vi "PoseAndTargeting.vi"() -> ()   [LabVIEW 2019]
doc: "This VI manages the robot's pose (position, heading, and velocity) and targeting information. Data from the IMU, swerve drive encoders, swerve azimuth encoders, LimeLight, and LIDAR are fused together to estimate these values. Supports pose resets on boot, from the Autonomous Sequencer, and on command from the FRC 4265 Dashboard."
uses:
  dsinstructions.vi
  sensors.vi
  dsdata.vi
  outputs.vi
  constants.vi
  autoninfo.vi
panel:
  out "Y Position (in)":dbl
  out "X Position (in)":dbl
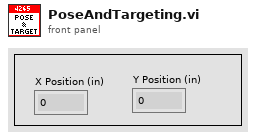
[diagram p1: front panel]
types:
  T1 = enum16{"Center", "North", "NorthWest", "West", "SouthWest", "South", "SouthEast", "East", "NorthEast"}
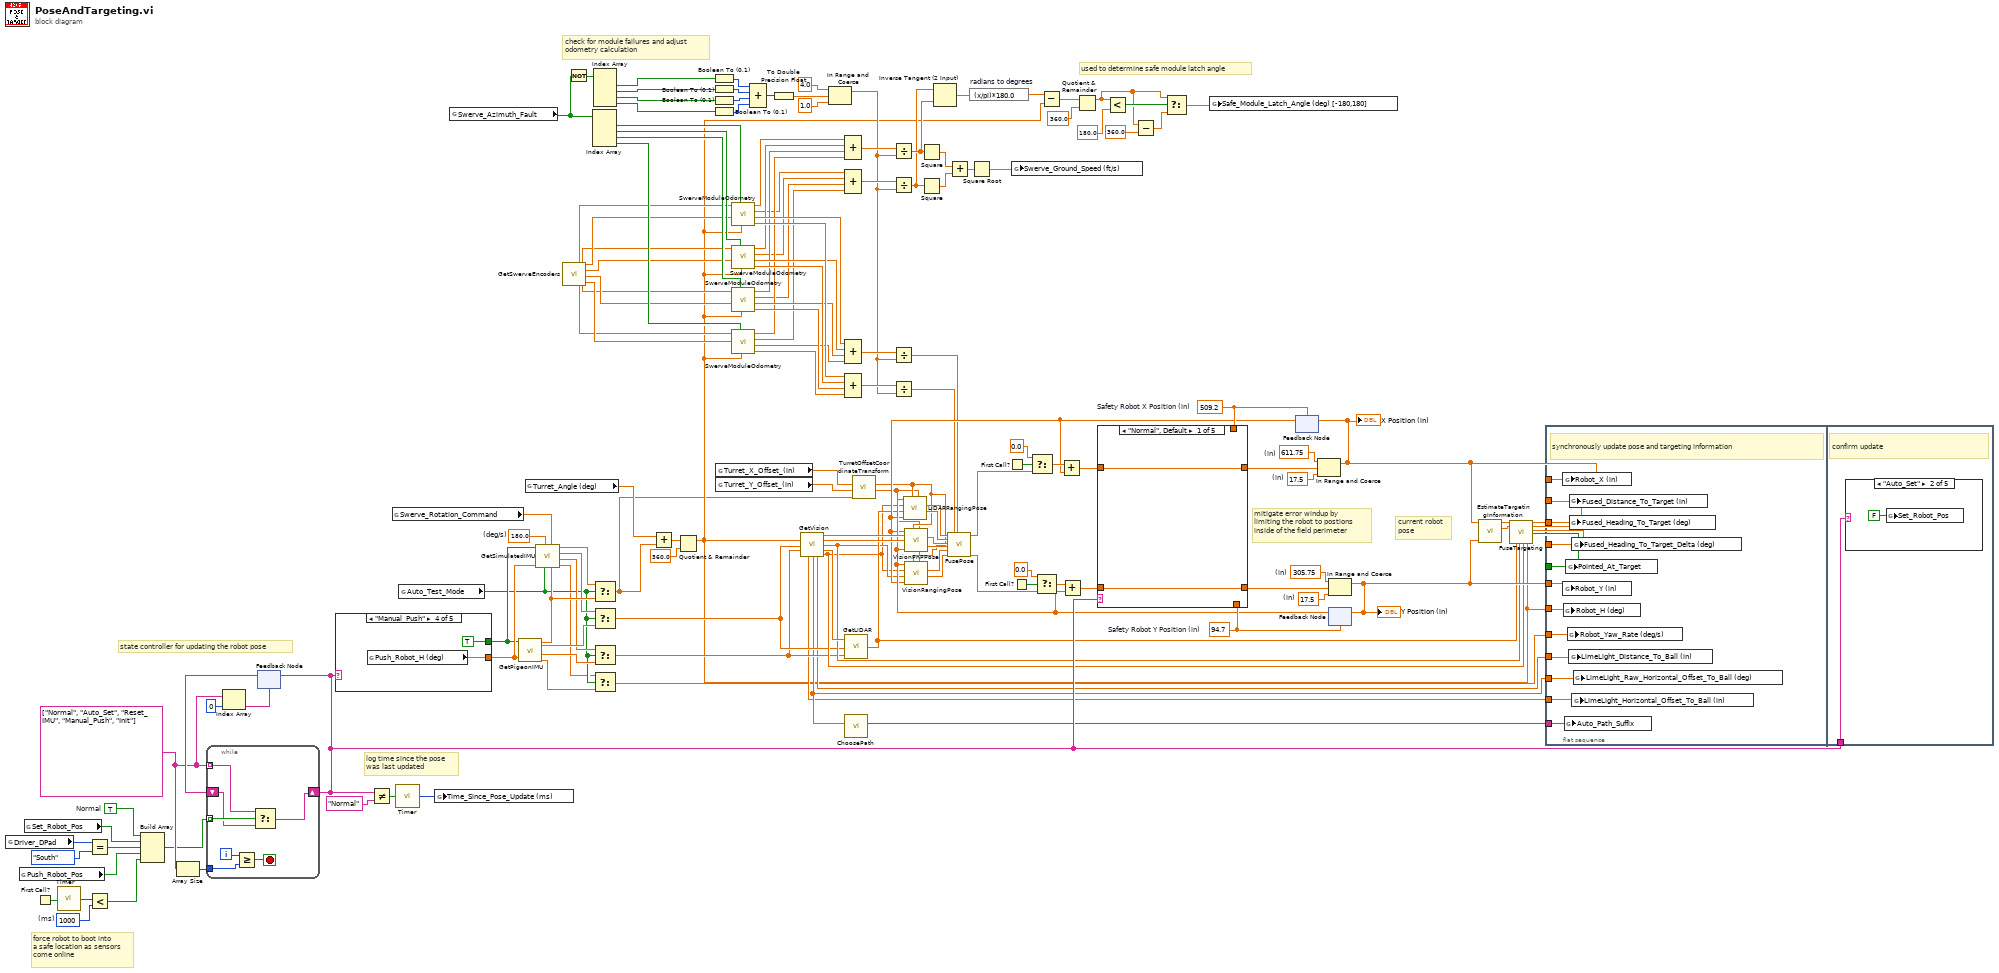
[diagram p0: block diagram]
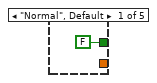
[diagram p6: hidden frame]
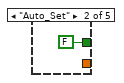
[diagram p7: hidden frame]
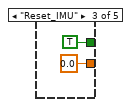
[diagram p8: hidden frame]
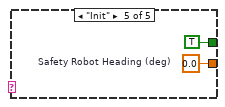
[diagram p9: hidden frame]
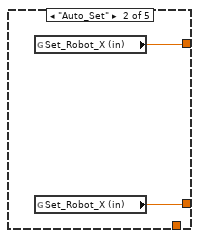
[diagram p10: hidden frame]
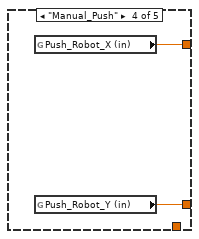
[diagram p12: hidden frame]
diagram:
  w94 = 180.0  # (deg/s)
  w98 = u32 1000  # (ms)
  w116 = string[] ["Normal", "Auto_Set", "Reset_IMU", "Manual_Push", "Init"] ("State Names")
  w115 = TRUE  # Normal
  w125 = 305.75  # (in)
  w126 = 17.5  # (in)
  w130 = 611.75  # (in)
  w131 = 17.5  # (in)
  w103 = 509.2  # Safety Robot X Position (in)
  w102 = 94.7  # Safety Robot Y Position (in)
  # "used to determine safe module latch angle"
  # "force robot to boot into\na safe location as sensors\ncome online"
  # "log time since the pose\nwas last updated"
  # "state controller for updating the robot pose"
  # "current robot\npose"
  # "mitigate error windup by\nlimiting the robot to postions\ninside of the field perimeter"
  # "check for module failures and adjust\nodometry calculation"
  n1 = global read "dsinstructions.vi" "Driver_DPad"() -> (w133:T1)
  n2 = global read "sensors.vi" "Push_Robot_Pos"() -> (w117:bool)
  n3 = global read "sensors.vi" "Set_Robot_Pos"() -> (w93:bool)
  n4 = First Call?() -> (First Call?: T/F=w101:bool)
  n5 = call "Timer.vi"("Reset Timer"=w101) -> ("Time (ms)"=w100:u32)
  n6 = Equal?(x=w133, y=T1."South") -> (x = y?=w92:bool)
  n7 = Less?(x=w100, y=w98) -> (x < y?=w99:bool)
  n8 = Build Array(w115, w93, w92, w117, w99) -> (w114:bool[])
  n9 = Array Size(array=w116) -> (size(s)=w118:i32)
  n10 = Index Array(array=w116, index=0) -> (element=w120:string)
  n11 = feedback #1(w120) -> (w119:string)
  n12 = while {
    tunnel: w114 -> [w161] mode=indexing
    tunnel: w116 -> [w159] mode=indexing
    shift-right: [w158] -> w107
    shift-left: w119 -> [w160]
    tunnel: w118 -> [w156]
    i -> [w157]
    stop <- w155 stop-if-true
    n13 = Greater Or Equal?(x=w157, y=w156) -> (x >= y?=w155:bool)
    n14 = Select(t=w159, s=w161, f=w160) -> (s? t:f=w158:string)
  }
  n15 = feedback-in #1(w107) -> ()
  n16 = case shown="\"Manual_Push\"" w107 {
    tunnel: [_ _ 0.0 ("Push_Robot_H (deg)") w167 w168] -> w97
    tunnel: [FALSE FALSE TRUE TRUE TRUE] -> w96
    frame "Normal", Default {
    }
    frame "Auto_Set" {
    }
    frame "Reset_IMU" {
    }
    frame "Manual_Push" {
      n17 = global read "sensors.vi" "Push_Robot_H (deg)"() -> (w167:dbl)
    }
    frame "Init" {
      w168 = 0.0  # Safety Robot Heading (deg)
    }
  }
  n18 = Not Equal?(x=w107, y="Normal") -> (x != y?=w106:bool)
  n19 = global read "outputs.vi" "Swerve_Rotation_Command"() -> (w95:dbl)
  n20 = call "Timer.vi"("Reset Timer"=w106) -> ("Time (ms)"=w104:u32)
  n21 = global read "dsdata.vi" "Auto_Test_Mode"() -> (w25:bool)
  n22 = global write "sensors.vi" "Time_Since_Pose_Update (ms)"(w104) -> ()
  n23 = global read "sensors.vi" "Swerve_Azimuth_Fault"() -> (w148:bool[])
  n24 = call "GetPigeonIMU.vi"("Reset Yaw (deg)"=w97, "Reset Yaw"=w96) -> ("Yaw Rate (deg/s)"=w24:dbl, "Roll (deg)"=w55:dbl, "Pitch (deg)"=w57:dbl, "Yaw (deg)"=w59:dbl)  [unwired: 6 in]
  n25 = global read "sensors.vi" "Turret_Angle (deg)"() -> (w9:dbl)
  n26 = call "GetSimulatedIMU.vi"("Real IMU Yaw (deg)"=w59, "Rotation Command"=w95, "Auto Test Mode"=w25, "Max Simulated Rotation Speed (deg/s)"=w94, "Reset Yaw (deg)"=w97, "Reset Yaw"=w96) -> ("Simulated Yaw Rate (deg/s)"=w23:dbl, "Simulated Roll (deg)"=w56:dbl, "Simulated Pitch (deg)"=w58:dbl, "Simulated Yaw (deg)"=w60:dbl)  [unwired: 2 in]
  n27 = call "GetSwerveEncoders.vi"() -> ("Swerve 0 Velocity (ft/s)"=w33:dbl, "Swerve 3 Velocity (ft/s)"=w30:dbl, "Swerve 1 Velocity (ft/s)"=w32:dbl, "Swerve 2 Velocity (ft/s)"=w31:dbl, "Swerve 0 Azimuth Position (deg)"=w91:dbl, "Swerve 1 Azimuth Position (deg)"=w90:dbl, "Swerve 2 Azimuth Position (deg)"=w89:dbl, "Swerve 3 Azimuth Position (deg)"=w88:dbl)  [unwired: 20 in]
  n28 = Not(x=w148) -> (.not. x?=w147:bool[])
  n29 = Index Array(array=w148) -> (element #1=w137:bool, element #2=w136:bool, element #3=w135:bool, element #4=w134:bool)  [unwired: 4 in]
  n30 = Index Array(array=w147) -> (element #1=w146:bool, element #2=w145:bool, element #3=w144:bool, element #4=w143:bool)  [unwired: 4 in]
  n31 = Select(t=w60, s=w25, f=w59) -> (s? t:f=w3:dbl)
  n32 = Select(t=w58, s=w25, f=w57) -> (s? t:f=w54:dbl)
  n33 = Select(t=w56, s=w25, f=w55) -> (s? t:f=w53:dbl)
  n34 = Select(t=w23, s=w25, f=w24) -> (s? t:f=w22:dbl)
  n35 = Add(x=w9, y=w3) -> (x+y=w8:dbl)
  n36 = Quotient & Remainder(x=w8, y=360.0) -> (x-y*floor(x/y)=w6:dbl)  [unwired: 1 out]
  n37 = Boolean To (0,1)(Boolean=w146) -> (0, 1=w142:i16)
  n38 = Boolean To (0,1)(Boolean=w145) -> (0, 1=w141:i16)
  n39 = Boolean To (0,1)(Boolean=w144) -> (0, 1=w140:i16)
  n40 = Boolean To (0,1)(Boolean=w143) -> (0, 1=w139:i16)
  n41 = global read "constants.vi" "Turret_X_Offset_(in)"() -> (w5:dbl)
  n42 = global read "constants.vi" "Turret_Y_Offset_(in)"() -> (w4:dbl)
  n43 = call "SwerveModuleOdometry.vi"("Robot Heading(deg)"=w6, "Module Fault"=w137, "Wheel Azimuth (deg)"=w91, "Velocity (ft/s)"=w33) -> ("Delta Y (in)"=w149:dbl, "Delta X (in)"=w52:dbl, "Velocity Y (ft/s)"=w44:dbl, "Velocity X (ft/s)"=w48:dbl)  [unwired: 2 in]
  n44 = call "SwerveModuleOdometry.vi"("Robot Heading(deg)"=w6, "Module Fault"=w136, "Wheel Azimuth (deg)"=w90, "Velocity (ft/s)"=w32) -> ("Delta Y (in)"=w150:dbl, "Delta X (in)"=w51:dbl, "Velocity Y (ft/s)"=w43:dbl, "Velocity X (ft/s)"=w47:dbl)  [unwired: 2 in]
  n45 = call "SwerveModuleOdometry.vi"("Robot Heading(deg)"=w6, "Module Fault"=w135, "Wheel Azimuth (deg)"=w89, "Velocity (ft/s)"=w31) -> ("Delta Y (in)"=w151:dbl, "Delta X (in)"=w50:dbl, "Velocity Y (ft/s)"=w42:dbl, "Velocity X (ft/s)"=w46:dbl)  [unwired: 2 in]
  n46 = call "SwerveModuleOdometry.vi"("Robot Heading(deg)"=w6, "Module Fault"=w134, "Wheel Azimuth (deg)"=w88, "Velocity (ft/s)"=w30) -> ("Delta Y (in)"=w152:dbl, "Delta X (in)"=w49:dbl, "Velocity Y (ft/s)"=w41:dbl, "Velocity X (ft/s)"=w45:dbl)  [unwired: 2 in]
  n47 = Compound Arithmetic op=ADD(w142, w141, w140, w139) -> (w138:i16)
  n48 = To Double Precision Float(number=w138) -> (double precision float=w83:dbl)
  n49 = call "GetVision.vi"("Turret_H (deg)"=w6, "Pitch (deg)"=w54, "Roll (deg)"=w53) -> ("LimeLight Raw Z Power Port (in)"=w87:dbl, "LimeLight Raw X Power Port (in)"=w86:dbl, "LimeLight Distance to Power Port (in)"=w66:dbl, "LimeLight Raw Horizontal Offset Power Port (deg)"=w68:dbl, "LimeLight Horizontal Offset to Ball (in)"=w26:dbl, "LimeLight Raw Horizontal Offset to Ball (deg)"=w28:dbl, "LimeLight Distance to Ball (in)"=w29:dbl, "LimeLight Heading to Power Port (deg)"=w61:dbl)  [unwired: 5 in]
  n50 = In Range and Coerce(upper limit=4.0, x=w83, lower limit=1.0) -> (coerced(x)=w38:dbl)  [unwired: 1 out]
  n51 = Compound Arithmetic op=ADD(w48, w47, w46, w45) -> (w40:dbl)
  n52 = Compound Arithmetic op=ADD(w44, w43, w42, w41) -> (w39:dbl)
  n53 = Compound Arithmetic op=ADD(w52, w51, w50, w49) -> (w154:dbl)
  n54 = Compound Arithmetic op=ADD(w149, w150, w151, w152) -> (w153:dbl)
  n55 = call "GetLIDAR.vi"("Roll (deg)"=w53, "Pitch (deg)"=w54, "Raw Horizontal Offset (in)"=w68) -> ("LIDAR Distance to Target (in)"=w67:dbl)
  n56 = call "ChoosePath.vi"("Limelight Raw Horizontal Offset to Ball (deg)"=w28) -> ("Auto Path Suffix"=w27:string)  [unwired: 10 in]
  n57 = call "TurretOffsetCoordinateTransform.vi"("Robot_Heading_(deg)"=w3, "Turret_Y_Offset_(in)"=w4, "Turret_X_Offset_(in)"=w5) -> ("Turret_Delta_Y"=w1:dbl, "Turret_Delta_X"=w2:dbl)  [unwired: 7 in]
  n58 = Divide(x=w40, y=w38) -> (x/y=w21:dbl)
  n59 = Divide(x=w39, y=w38) -> (x/y=w20:dbl)
  n60 = Divide(x=w154, y=w38) -> (x/y=w78:dbl)
  n61 = Divide(x=w153, y=w38) -> (x/y=w77:dbl)
  n62 = Square(x=w21) -> (x^2=w36:dbl)
  n63 = Square(x=w20) -> (x^2=w37:dbl)
  n64 = Inverse Tangent (2 Input)(1:w21, 2:w20) -> (0:w19:dbl)
  n65 = Add(x=w36, y=w37) -> (x+y=w35:dbl)
  n66 = expression code="(x/pi)*180.0" "radians to degrees"(w19) -> (w18:dbl)
  n67 = Square Root(x=w35) -> (sqrt(x)=w34:dbl)
  n68 = First Call?() -> (First Call?: T/F=w128:bool)
  n69 = First Call?() -> (First Call?: T/F=w123:bool)
  n70 = global write "sensors.vi" "Swerve_Ground_Speed (ft/s)"(w34) -> ()
  n71 = Subtract(x=w18, y=w6) -> (x-y=w11:dbl)
  n72 = Quotient & Remainder(x=w11, y=360.0) -> (x-y*floor(x/y)=w14:dbl)  [unwired: 1 out]
  n73 = Less?(x=w14, y=180.0) -> (x < y?=w15:bool)
  n74 = Subtract(x=w14, y=360.0) -> (x-y=w13:dbl)
  n75 = Select(t=w14, s=w15, f=w13) -> (s? t:f=w10:dbl)
  n76 = global write "sensors.vi" "Safe_Module_Latch_Angle (deg) [-180,180]"(w10) -> ()
  n77 = feedback #2(w103) -> (w84:dbl)
  n78 = feedback #3(w102) -> (w85:dbl)
  n79 = call "LIDARRangingPose.vi"("Turret Delta Y"=w1, "Turret Delta X"=w2, "Previous X Position (in)"=w84, "Distance to Target (in)"=w67, "Heading to Target (deg)"=w61, "Previous Y Position (in)"=w85) -> ("Delta Y (in)"=w75:dbl, "Delta X (in)"=w76:dbl)  [unwired: 4 in]
  n80 = call "VisionPnPPose.vi"("Turret Delta Y"=w1, "Turret Delta X"=w2, "Previous Y Estimate (in)"=w85, "LimeLight Raw X (in)"=w86, "LimeLight Raw Z (in)"=w87, "Previous X Estimate (in)"=w84) -> ("deltaY (in)"=w73:dbl, "deltaX (in)"=w74:dbl)  [unwired: 4 in]
  n81 = call "VisionRangingPose.vi"("Turret Delta Y"=w1, "Turret Delta X"=w2, "Previous X Position (in)"=w84, "Distance to Target (in)"=w66, "Heading to Target (deg)"=w61, "Previous Y Position (in)"=w85) -> ("Delta Y (in)"=w71:dbl, "Delta X (in)"=w72:dbl)  [unwired: 4 in]
  n82 = call "FusePose.vi"("LIDAR range deltaX"=w76, "LIDAR range deltaY"=w75, "LimeLight PnP deltaX"=w74, "LimeLight PnP deltaY"=w73, "LimeLight range deltaX"=w72, "LimeLight range deltaY"=w71, "Odometry deltaY"=w77, "Odometry deltaX"=w78) -> ("Fused deltaX"=w80:dbl, "Fused deltaY"=w79:dbl)  [unwired: 10 in]
  n83 = Select(t=0.0, s=w128, f=w80) -> (s? t:f=w129:dbl)
  n84 = Select(t=0.0, s=w123, f=w79) -> (s? t:f=w124:dbl)
  n85 = Add(x=w129, y=w84) -> (x+y=w113:dbl)
  n86 = Add(x=w124, y=w85) -> (x+y=w111:dbl)
  n87 = case shown="\"Normal\", Default" w107 {
    tunnel: w113 -> [w171 _ w175 _ _]
    tunnel: [w171 w173 w175 w177 w179] -> w112
    tunnel: w111 -> [w170 _ w174 _ _]
    tunnel: [w170 w172 w174 w176 w178] -> w110
    tunnel: w103 -> [_ _ _ _ w179]
    tunnel: w102 -> [_ _ _ _ w178]
    frame "Normal", Default {
    }
    frame "Auto_Set" {
      n88 = global read "sensors.vi" "Set_Robot_X (in)"() -> (w173:dbl)
      n89 = global read "sensors.vi" "Set_Robot_X (in)"() -> (w172:dbl)
    }
    frame "Reset_IMU" {
    }
    frame "Manual_Push" {
      n90 = global read "sensors.vi" "Push_Robot_X (in)"() -> (w177:dbl)
      n91 = global read "sensors.vi" "Push_Robot_Y (in)"() -> (w176:dbl)
    }
    frame "Init" {
    }
  }
  n92 = In Range and Coerce(upper limit=w130, x=w112, lower limit=w131) -> (coerced(x)=w109:dbl)  [unwired: 1 out]
  "X Position (in)" <- w109
  n93 = feedback-in #2(w109) -> ()
  n94 = In Range and Coerce(upper limit=w125, x=w110, lower limit=w126) -> (coerced(x)=w108:dbl)  [unwired: 1 out]
  "Y Position (in)" <- w108
  n95 = feedback-in #3(w108) -> ()
  n96 = call "EstimateTargetingInformation.vi"("Robot Y (in)"=w108, "Robot X (in)"=w109) -> ("Estimated Robot Heading to Target (deg)"=w69:dbl, "Estimated Distance to Target (in)"=w70:dbl)  [unwired: 7 in]
  n97 = call "FuseTargeting.vi"("Estimated Distance to Target (in)"=w70, "Estimated Heading to Target (deg)"=w69, "LIDAR Distance to Target (in)"=w67, "LimeLight Distance to Target (in)"=w66, "LimeLight Heading to Target (deg)"=w61, "Robot_H (deg)"=w6) -> ("Fused Distance to Target (in)"=w65:dbl, "Fused Heading to Target (deg)"=w64:dbl, "Fused Heading to Target Delta (deg)"=w63:dbl, "Pointed at Target"=w62:bool)  [unwired: 10 in]
  n98 = flat-sequence {
    tunnel: w109 -> [w191]
    tunnel: w108 -> [w190]
    tunnel: w6 -> [w189]
    tunnel: w65 -> [w188]
    tunnel: w64 -> [w187]
    tunnel: w63 -> [w186]
    tunnel: w62 -> [w185]
    tunnel: w29 -> [w184]
    tunnel: w28 -> [w183]
    tunnel: w27 -> [w182]
    tunnel: w26 -> [w181]
    tunnel: w22 -> [w180]
    tunnel: w107 -> [w192]
    frame #0 {
      # "synchronously update pose and targeting information"
      n99 = global write "sensors.vi" "Robot_X (in)"(w191) -> ()
      n100 = global write "sensors.vi" "Robot_Y (in)"(w190) -> ()
      n101 = global write "sensors.vi" "Robot_H (deg)"(w189) -> ()
      n102 = global write "autoninfo.vi" "Auto_Path_Suffix"(w182) -> ()
      n103 = global write "sensors.vi" "Pointed_At_Target"(w185) -> ()
      n104 = global write "sensors.vi" "Robot_Yaw_Rate (deg/s)"(w180) -> ()
      n105 = global write "sensors.vi" "LimeLight_Distance_To_Ball (in)"(w184) -> ()
      n106 = global write "sensors.vi" "Fused_Distance_To_Target (in)"(w188) -> ()
      n107 = global write "sensors.vi" "Fused_Heading_To_Target (deg)"(w187) -> ()
      n108 = global write "sensors.vi" "Fused_Heading_To_Target_Delta (deg)"(w186) -> ()
      n109 = global write "sensors.vi" "LimeLight_Horizontal_Offset_To_Ball (in)"(w181) -> ()
      n110 = global write "sensors.vi" "LimeLight_Raw_Horizontal_Offset_To_Ball (deg)"(w183) -> ()
    }
    frame #1 {
      # "confirm update"
      n111 = case shown="\"Auto_Set\"" w192 {
        frame "Normal", Default {
        }
        frame "Auto_Set" {
          n112 = global write "sensors.vi" "Set_Robot_Pos"(FALSE ("Set_Robot_Pos")) -> ()
        }
        frame "Reset_IMU" {
        }
        frame "Manual_Push" {
        }
        frame "Init" {
        }
      }
    }
  }
